vi "ADQ214 Get Gain And Offset.vi"(0 "adq_cu_ptr":u32, 1 "Offset":i32, 5 "adq212_num":i32, 7 "channel":u8, 9 "Gain":i32, 11 "error in (no error)":errorcluster) -> (3 "Offset out":i32, 4 "adq_cu_ptr out":u32, 6 "function return":u32, 10 "Gain out":i32, 15 "error out":errorcluster)   [LabVIEW 8.6, in "ADQAPI.lvlib"]
doc: "extern \"C\" __declspec(dllimport) unsigned int ADQ214_GetGainAndOffset(void* adq_cu_ptr, int adq212_num, unsigned char channel, int* Gain, int* Offset);"
uses:
  F/HRT/Sp Devices Thesis/ADQ-214 project (H R)/ADQAPI.lvlib
  F:/HRT/Sp Devices Thesis/ADQ-214 project (H R)/ADQAPI.dll
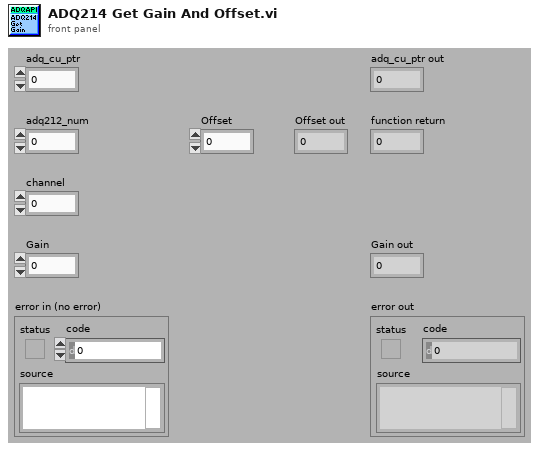
[diagram p1: front panel]
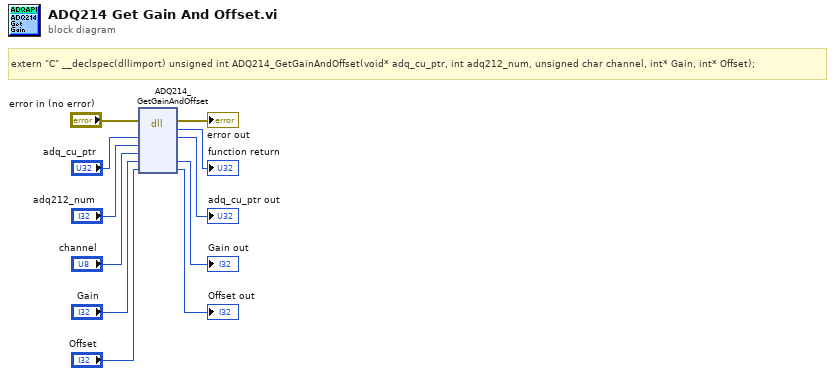
[diagram p0: block diagram]
diagram:
  # "extern \"C\" __declspec(dllimport) unsigned int\tADQ214_GetGainAndOffset(void* adq_cu_ptr, int adq212_num, unsigned char channel, int* Gain, int* Offset);"
  n1 = dll-call lib="F:/HRT/Sp Devices Thesis/ADQ-214 project (H R)/ADQAPI.*" fn="ADQ214_GetGainAndOffset"(error in="error in (no error)", "adq_cu_ptr"="adq_cu_ptr", "adq212_num"="adq212_num", "channel"="channel", "Gain"="Gain", "Offset"="Offset") -> (error out=→"error out":errorcluster, →"function return":u32, "adq_cu_ptr"=→"adq_cu_ptr out":u32, "Gain"=→"Gain out":i32, "Offset"=→"Offset out":i32)  [unwired: 4 in, 1 out]
